vi "Gait to Desired Theta v3.vi"(11 "Current Gait %":dbl) -> (2 "Current Desired Theta":dbl)   [LabVIEW 2018]
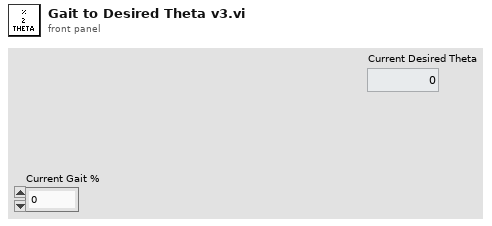
[diagram p1: front panel]
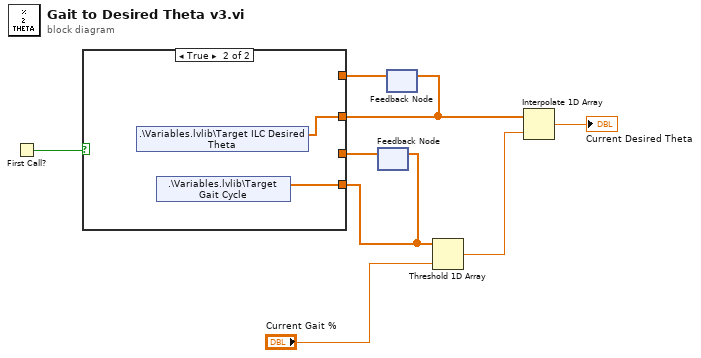
[diagram p0: block diagram]
diagram:
  n1 = First Call?() -> (First Call?: T/F=w5:bool)
  n2 = feedback #1() -> (w1:dbl[])  [unwired: 1 in]
  n3 = feedback #2() -> (w3:dbl[])  [unwired: 1 in]
  n4 = case shown="True" w5 {
    tunnel: [w10 w12] -> w4
    tunnel: [w9 w11] -> w2
    tunnel: w3 -> [w10 _]
    tunnel: w1 -> [w9 _]
    frame False {
    }
    frame True {
      n5 = shared-variable ".\\Variables.lvlib\\Target ILC Desired Theta"() -> (w12:dbl[])  [unwired: 1 in, 1 out]
      n6 = shared-variable ".\\Variables.lvlib\\Target Gait Cycle"() -> (w11:dbl[])  [unwired: 1 in, 1 out]
    }
  }
  n7 = feedback-in #1(w2) -> ()
  n8 = feedback-in #2(w4) -> ()
  n9 = Threshold 1D Array(2:"Current Gait %", 3:w2) -> (0:w7:dbl)  [unwired: 1 in]
  n10 = Interpolate 1D Array(1:w7, 2:w4) -> (0:→"Current Desired Theta":dbl)
